vi "Render Node.vi"(8 "Error In":errorcluster, 10 "Node":refnum<class "Node.lvclass">, 11 "Renderer In":refnum<class "Renderer.lvclass">) -> (0 "Error Out":errorcluster, 2 "Output":string, 3 "Renderer Out":refnum<class "Renderer.lvclass">)   [LabVIEW 2018, in "Toolkit.lvlib" / "Renderer.lvclass"]
uses:
  Renderer.lvclass
  Nodes/Node/Node.lvclass
  Nodes/Comment/Comment.lvclass
  Nodes/Delimiter/Delimiter.lvclass
  Nodes/Partial/Partial.lvclass
  Nodes/Section/Section.lvclass
  Nodes/Text/Text.lvclass
  Nodes/Variable/Variable.lvclass
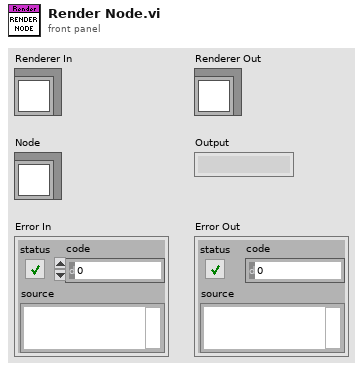
[diagram p1: front panel]
types:
  T1 = typedef "Toolkit.lvlib/Nodes.lvlib/Types.ctl" = enum16{"Comment", "Delimiter", "Partial", "Root", "Section", "Text", "Unknown", "Variable"}
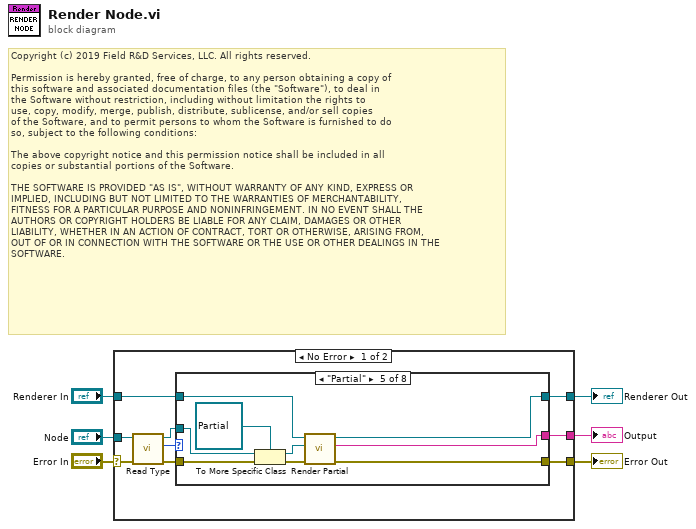
[diagram p0: block diagram]
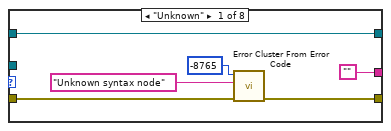
[diagram p2: hidden frame]
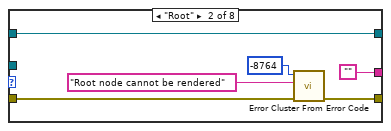
[diagram p3: hidden frame]
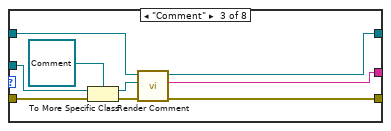
[diagram p4: hidden frame]
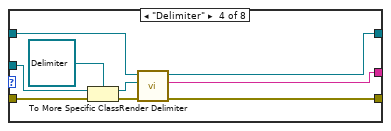
[diagram p5: hidden frame]
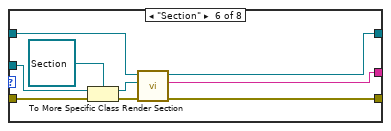
[diagram p6: hidden frame]
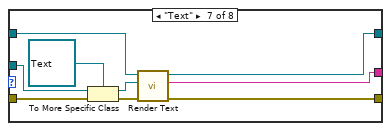
[diagram p7: hidden frame]
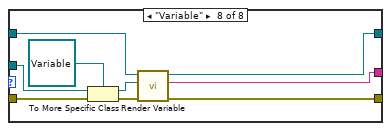
[diagram p8: hidden frame]
diagram:
  # "Copyright (c) 2019 Field R&D Services, LLC. All rights reserved.\n\nPermission is hereby granted, free of charge, to any person obtaining a copy of\nthis software and associated documentation files (the \"Software\"), to deal in\nthe Software without restriction, including without limitation the rights to\nuse, copy, modify, merge, publish, distribute, sublicense, and/or sell copies\nof the Software, and to permit persons to whom the Software is furnished to do\nso, subject to the following conditions:\n\nThe above copyright notice and this permission notice shall be included in all\ncopies or substantial portions of the Software.\n\nTHE SOFTWARE IS PROVIDED \"AS IS\", WITHOUT WARRANTY OF ANY KIND, EXPRESS OR\nIMPLIED, INCLUDING BUT NOT LIMITED TO THE WARRANTIES OF MERCHANTABILITY,\nFITNESS FOR A PARTICULAR PURPOSE AND NONINFRINGEMENT. IN NO EVENT SHALL THE\nAUTHORS OR COPYRIGHT HOLDERS BE LIABLE FOR ANY CLAIM, DAMAGES OR OTHER\nLIABILITY, WHETHER IN AN ACTION OF CONTRACT, TORT OR OTHERWISE, ARISING FROM,\nOUT OF OR IN CONNECTION WITH THE SOFTWARE OR THE USE OR OTHER DEALINGS IN THE\nSOFTWARE."
  n1 = case shown="No Error" "Error In" {
    selector: "Error In" -> [w9 w82]
    tunnel: [w10 w83] -> w1
    tunnel: "Renderer In" -> [w7 w83]
    tunnel: [w12 _] -> w6
    tunnel: "Node" -> [w8 _]
    tunnel: [w11 w82] -> w4
    frame No Error {
      n2 = call-dynamic "Read Type.vi"("Error In"=w9, "Node In"=w8) -> ("Error Out"=w13:errorcluster, "Type"=w14:T1, "Node Out"=w15:refnum<class "Node.lvclass">)  [unwired: 7 in]
      n3 = case shown="\"Partial\"" w14 {
        tunnel: w13 -> [w19 w23 w36 w45 w54 w63 w71 w79]
        tunnel: [w18 w22 w35 w44 w47 w62 w65 w74] -> w11
        tunnel: w15 -> [_ _ w33 w42 w53 w60 w72 w80]
        tunnel: ["" "" w30 w40 w48 w58 w67 w75] -> w12
        tunnel: w7 -> [w21 w27 w28 w37 w50 w56 w64 w73]
        tunnel: [w21 w27 w29 w39 w49 w55 w66 w76] -> w10
        frame "Unknown" {
          n4 = call <vilib>:"Error Cluster From Error Code.vi"("error in (no error)"=w19, "error message (\"\")"="Unknown syntax node" ("error message (\"\")"), "error code (0)"=-8765) -> ("error out"=w18:errorcluster)  [unwired: 6 in]
        }
        frame "Root" {
          n5 = call <vilib>:"Error Cluster From Error Code.vi"("error in (no error)"=w23, "error message (\"\")"="Root node cannot be rendered" ("error message (\"\")"), "error code (0)"=-8764) -> ("error out"=w22:errorcluster)  [unwired: 6 in]
        }
        frame "Comment" {
          n6 = To More Specific Class(target class=refnum<class "Comment.lvclass"> refnum ("Toolkit.lvlib:Nodes.lvlib:Comment.lvclass"), reference=w33, error in=w36) -> (specific class reference=w31:refnum<class "Comment.lvclass">, error out=w34:errorcluster)
          n7 = call "Render Comment.vi"("Error In"=w34, "Comment"=w31, "Renderer In"=w28) -> ("Error Out"=w35:errorcluster, "Output"=w30:string, "Renderer Out"=w29:refnum<class "Renderer.lvclass">)  [unwired: 6 in]
        }
        frame "Delimiter" {
          n8 = To More Specific Class(target class=refnum<class "Delimiter.lvclass"> refnum ("Toolkit.lvlib:Nodes.lvlib:Delimiter.lvclass"), reference=w42, error in=w45) -> (specific class reference=w41:refnum<class "Delimiter.lvclass">, error out=w43:errorcluster)
          n9 = call "Render Delimiter.vi"("Error In"=w43, "Delimiter"=w41, "Renderer In"=w37) -> ("Error Out"=w44:errorcluster, "Output"=w40:string, "Renderer Out"=w39:refnum<class "Renderer.lvclass">)  [unwired: 6 in]
        }
        frame "Partial" {
          n10 = To More Specific Class(target class=refnum<class "Partial.lvclass"> refnum ("Toolkit.lvlib:Nodes.lvlib:Partial.lvclass"), reference=w53, error in=w54) -> (specific class reference=w46:refnum<class "Partial.lvclass">, error out=w51:errorcluster)
          n11 = call "Render Partial.vi"("Error In"=w51, "Partial"=w46, "Renderer In"=w50) -> ("Error Out"=w47:errorcluster, "Output"=w48:string, "Renderer Out"=w49:refnum<class "Renderer.lvclass">)  [unwired: 6 in]
        }
        frame "Section" {
          n12 = To More Specific Class(target class=refnum<class "Section.lvclass"> refnum ("Toolkit.lvlib:Nodes.lvlib:Section.lvclass"), reference=w60, error in=w63) -> (specific class reference=w59:refnum<class "Section.lvclass">, error out=w61:errorcluster)
          n13 = call "Render Section.vi"("Error In"=w61, "Section"=w59, "Renderer In"=w56) -> ("Error Out"=w62:errorcluster, "Output"=w58:string, "Renderer Out"=w55:refnum<class "Renderer.lvclass">)  [unwired: 6 in]
        }
        frame "Text" {
          n14 = To More Specific Class(target class=refnum<class "Text.lvclass"> refnum ("Toolkit.lvlib:Nodes.lvlib:Text.lvclass"), reference=w72, error in=w71) -> (specific class reference=w68:refnum<class "Text.lvclass">, error out=w69:errorcluster)
          n15 = call "Render Text.vi"("Error In"=w69, "Text"=w68, "Renderer In"=w64) -> ("Error Out"=w65:errorcluster, "Content"=w67:string, "Renderer Out"=w66:refnum<class "Renderer.lvclass">)  [unwired: 6 in]
        }
        frame "Variable" {
          n16 = To More Specific Class(target class=refnum<class "Variable.lvclass"> refnum ("Toolkit.lvlib:Nodes.lvlib:Tag.lvclass"), reference=w80, error in=w79) -> (specific class reference=w77:refnum<class "Variable.lvclass">, error out=w78:errorcluster)
          n17 = call "Render Variable.vi"("Error In"=w78, "Tag"=w77, "Renderer In"=w73) -> ("Error Out"=w74:errorcluster, "Output"=w75:string, "Renderer Out"=w76:refnum<class "Renderer.lvclass">)  [unwired: 6 in]
        }
      }
    }
    frame Error {
    }
  }
  "Output" <- w6
  "Error Out" <- w4
  "Renderer Out" <- w1
